vi "Create Notifiers.vi"(8 "error in":errorcluster) -> (0 "error out":errorcluster, 3 "Notifiers":T1)   [LabVIEW 2015, in "Notifiers.lvlib"]
doc: "Creates notifiers for handshaking and closing processes"
uses:
  Notifiers.lvlib
  Notifiers.ctl
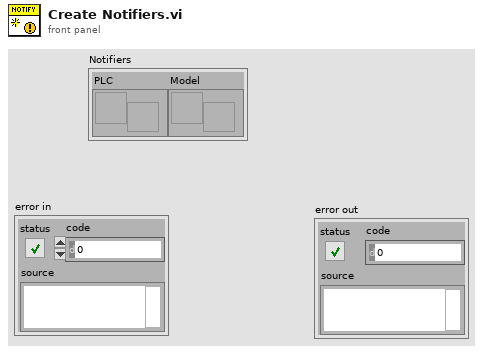
[diagram p1: front panel]
types:
  T1 = typedef "Notifiers.lvlib/Notifiers.ctl" = cluster{"PLC":refnum<notifier>, "Model":refnum<notifier>}
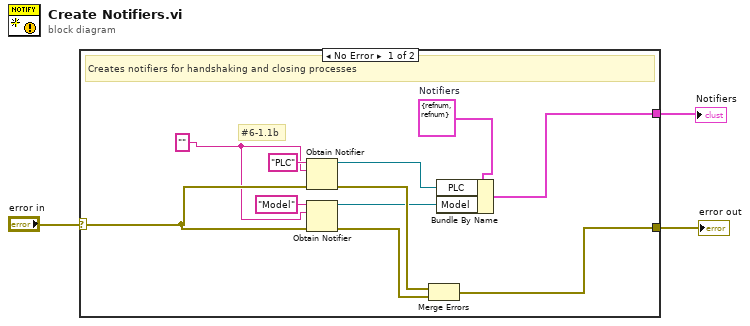
[diagram p0: block diagram]
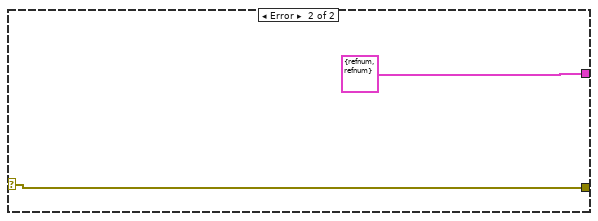
[diagram p2: hidden frame]
diagram:
  n1 = case shown="No Error" "error in" {
    selector: "error in" -> [w10 w16]
    tunnel: [w13 w16] -> w3
    tunnel: [w12 T1 {"PLC"=refnum, "Model"=refnum} ("Notifiers")] -> w2
    frame No Error {
      w6 = ""
      w9 = T1 {"PLC"=refnum, "Model"=refnum}  # Notifiers
      # "#6-1.1b"
      # "Creates notifiers for handshaking and closing processes"
      n2 = Obtain Notifier(name (unnamed)="PLC", notification data type=w6, error in (no error)=w10) -> (notifier out=w5:refnum<notifier>, error out=w14:errorcluster)  [unwired: 1 in, 1 out]
      n3 = Obtain Notifier(name (unnamed)="Model", notification data type=w6, error in (no error)=w10) -> (notifier out=w4:refnum<notifier>, error out=w11:errorcluster)  [unwired: 1 in, 1 out]
      n4 = Merge Errors(w14, w11) -> (w13:errorcluster)
      n5 = Bundle By Name(cluster=w9, "PLC"=w5, "Model"=w4) -> (w12:T1)
    }
    frame Error {
    }
  }
  "error out" <- w3
  "Notifiers" <- w2
